vi "X_2.84_Event_Structures.vi"() -> ()   [LabVIEW 2022 SP3]
uses:
  <vilib>/numeric/Random Number (Range) DBL.vi
panel:
  in  "stop":bool
  out "Log":string
  in  "Tab Control":enum32{"Page 1", "Page 2"}(tab)
  in  "Cluster 2":T1
  in  "Cluster":T2
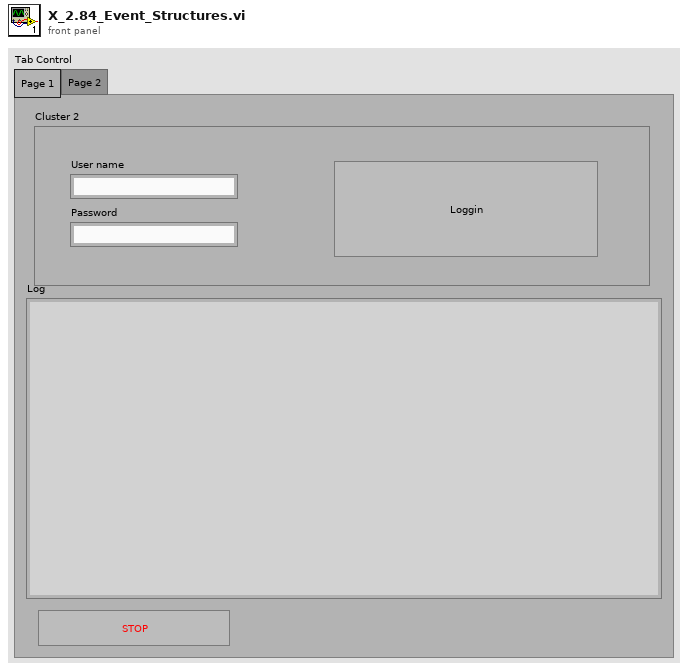
[diagram p1: front panel]
types:
  T1 = cluster{"User name":string, "Password":string, "Loggin":bool}
  T2 = cluster{"Generer Lille":bool, "Generer Stor":bool, "Multiply":bool, "Log af":bool}
  T3 = enum8{"Enabled", "Disabled", "Disabled and Grayed Out"}
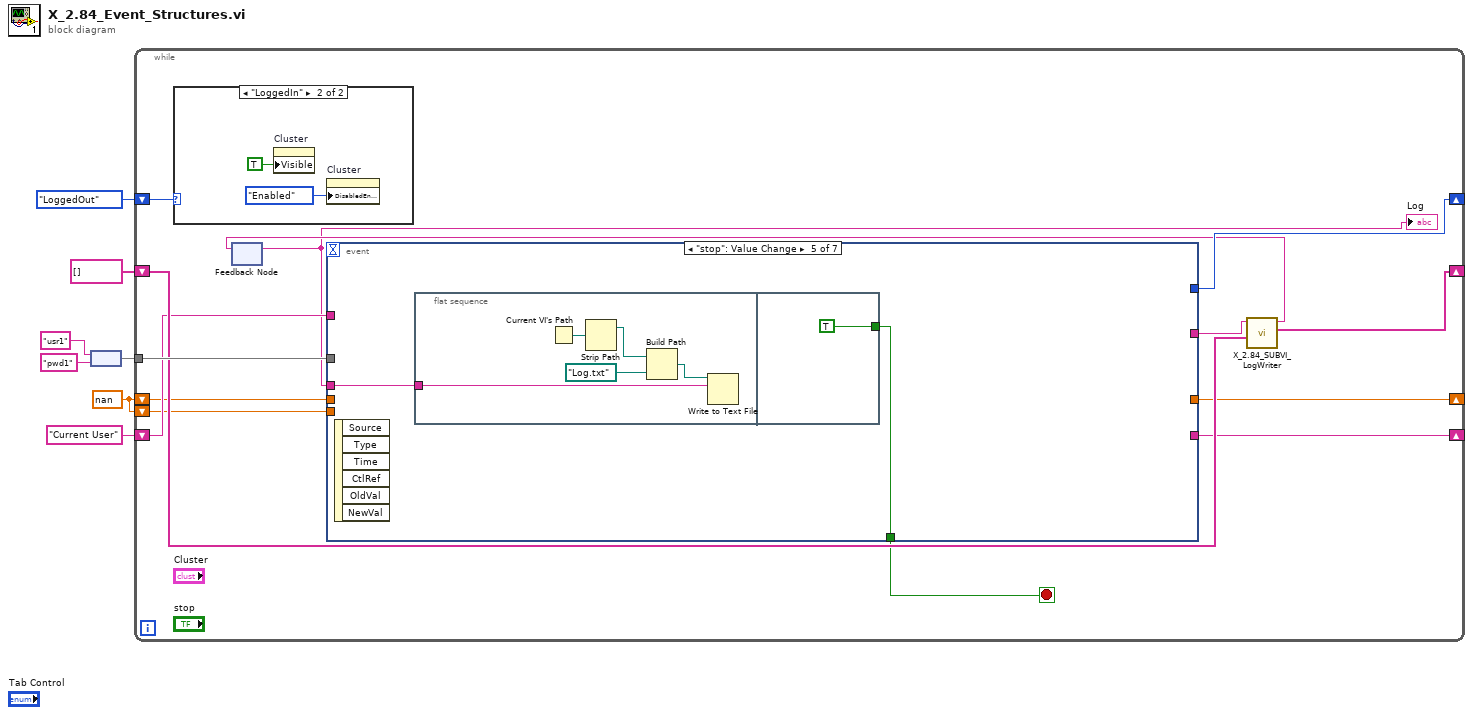
[diagram p0: block diagram]
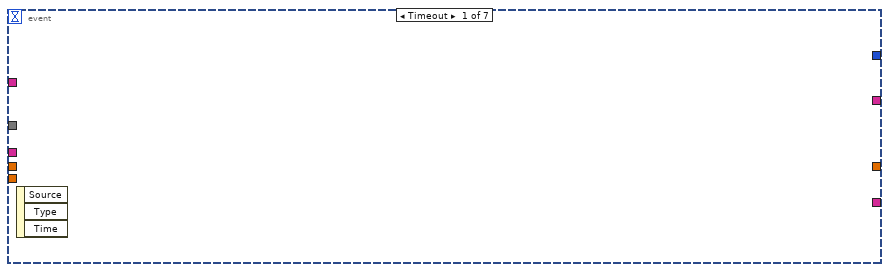
[diagram p2: hidden frame]
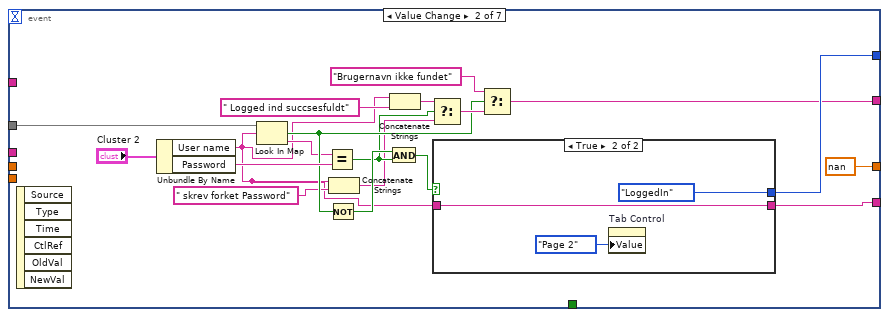
[diagram p3: hidden frame]
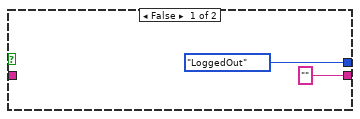
[diagram p4: hidden frame]
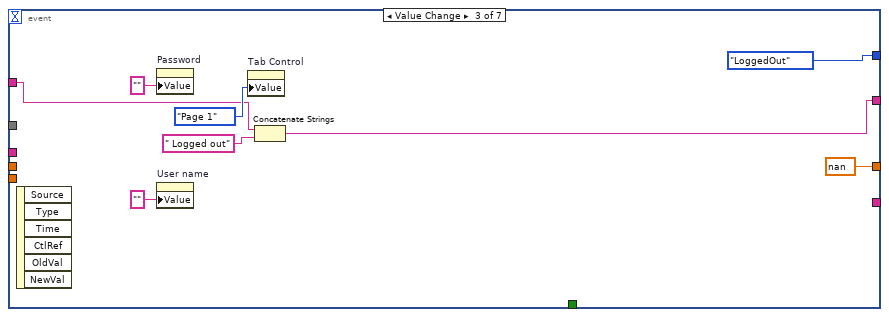
[diagram p5: hidden frame]
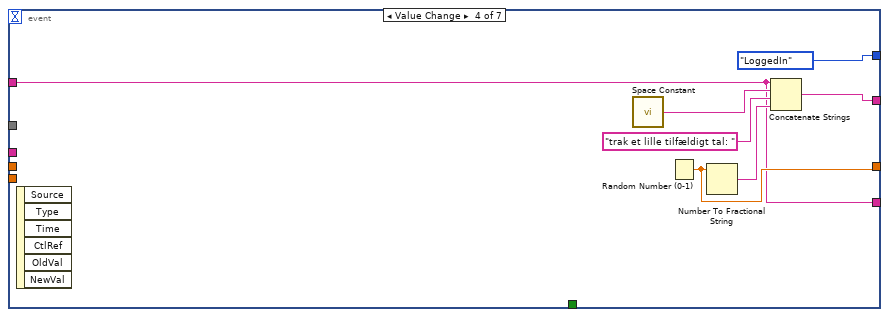
[diagram p6: hidden frame]
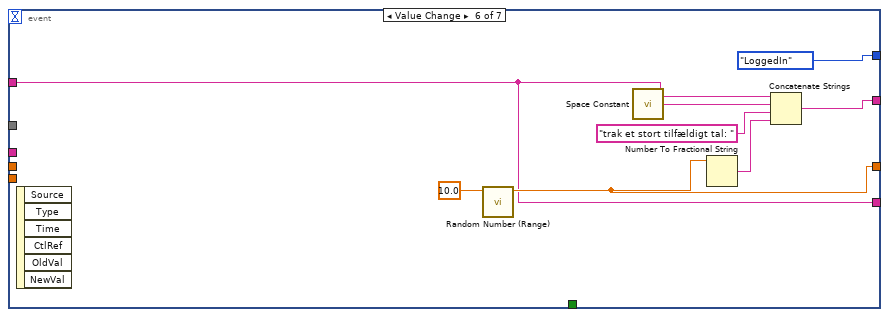
[diagram p7: hidden frame]
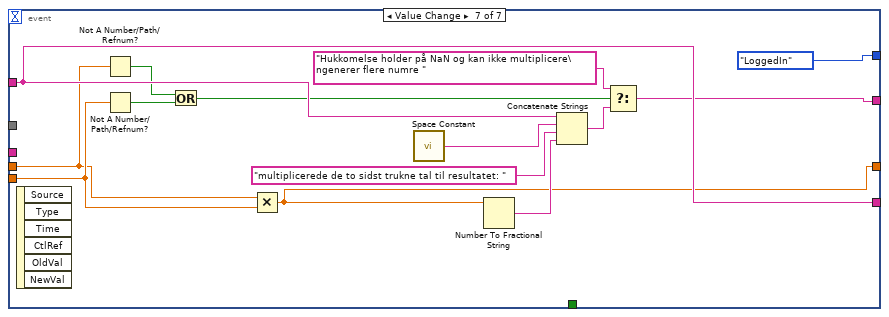
[diagram p8: hidden frame]
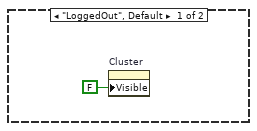
[diagram p9: hidden frame]
diagram:
  w2 = nan
  n1 = node("usr1" ("key"), "pwd1" ("key")) -> (w4:map{string, string})
  n2 = while {
    shift-right: [w19] -> _
    shift-left: enum16{"LoggedOut", "LoggedIn"}."LoggedOut" -> [w20]
    tunnel: w4 -> [w21]
    shift-right: [w17] -> _
    shift-left: string[] [] -> [w18]
    shift-right: [w15] -> _
    shift-left: w2 -> [w11]
    shift-left: w2 -> [w12]
    shift-right: [w14] -> _
    shift-left: "Current User" -> [w13]
    stop <- w10 stop-if-true
    n3 = case shown="\"LoggedIn\"" w20 {
      frame "LoggedOut", Default {
        n4 = property on="Cluster" class="Clust"("Visible"=FALSE) -> ()  [unwired: 2 in, 2 out]
      }
      frame "LoggedIn" {
        n5 = property on="Cluster" class="Clust"("Visible"=TRUE) -> ()  [unwired: 2 in, 2 out]
        n6 = property on="Cluster" class="Clust"("DisabledEnum"=T3."Enabled" ("Disabled")) -> ()  [unwired: 2 in, 2 out]
      }
    }
    n7 = feedback #1() -> (w8:string)  [unwired: 1 in]
    "Log" <- w8
    n8 = event shown="[4] \"stop\": Value Change" {
      selector: _ -> [_ _ _ _ _ _ _]
      dyn-events: _ -> [_ _ _ _ _ _ _]
      timeout: _ -> [_ _ _ _ _ _ _]
      tunnel: w21 -> [_ w40 _ _ _ _ _]
      tunnel: [_ w36 enum16{"LoggedOut", "LoggedIn"}."LoggedOut" enum16{"LoggedOut", "LoggedIn"}."LoggedIn" _ enum16{"LoggedOut", "LoggedIn"}."LoggedIn" enum16{"LoggedOut", "LoggedIn"}."LoggedIn"] -> w19
      tunnel: [_ w35 w46 w55 _ w70 w82] -> w16
      tunnel: [_ nan nan w59 _ w71 w81] -> w15
      tunnel: [_ w29 _ w54 _ w69 w85] -> w14
      tunnel: w13 -> [_ _ w48 w54 _ w69 w85]
      tunnel: w12 -> [_ _ _ _ _ _ w83]
      tunnel: w11 -> [_ _ _ _ _ _ w80]
      tunnel: [_ _ _ _ w62 _ _] -> w10
      tunnel: w8 -> [_ _ _ _ w61 _ _]
      event Timeout {
        n9 = event-data() -> ()  [unwired: 1 in, 3 out]
      }
      event "Cluster 2.Loggin": Value Change {
        n10 = event-data() -> ()  [unwired: 1 in, 6 out]
        n11 = Unbundle By Name("Cluster 2") -> ("User name"=w22:string, "Password"=w39:string)
        n12 = Look In Map(map=w40, key=w22) -> (key not found?=w34:bool, value=w28:string)  [unwired: 1 in]
        n13 = Equal?(x=w28, y=w39) -> (x = y?=w32:bool)
        n14 = Not(x=w34) -> (.not. x?=w33:bool)
        n15 = Concatenate Strings(w22, " skrev forket Password") -> (w25:string)
        n16 = And(x=w33, y=w32) -> (x .and. y?=w31:bool)
        n17 = Concatenate Strings(w22, " Logged ind succsesfuldt") -> (w23:string)
        n18 = Select(t=w23, s=w32, f=w25) -> (s? t:f=w37:string)
        n19 = case shown="True" w31 {
          tunnel: [enum16{"LoggedOut", "LoggedIn"}."LoggedOut" enum16{"LoggedOut", "LoggedIn"}."LoggedIn"] -> w36
          tunnel: w22 -> [_ w43]
          tunnel: ["" ("value") w43] -> w29
          frame False {
          }
          frame True {
            n20 = property on="Tab Control" class="TabCtl (strict)"("Value"=enum32{"Page 1", "Page 2"}."Page 2" ("Tab Control")) -> ()  [unwired: 2 in, 2 out]
          }
        }
        n21 = Select(t="Brugernavn ikke fundet", s=w34, f=w37) -> (s? t:f=w35:string)
      }
      event "Cluster.Log af": Value Change {
        n22 = event-data() -> ()  [unwired: 1 in, 6 out]
        n23 = property on="Password" class="Str"("Value"="") -> ()  [unwired: 2 in, 2 out]
        n24 = property on="User name" class="Str"("Value"="") -> ()  [unwired: 2 in, 2 out]
        n25 = property on="Tab Control" class="TabCtl (strict)"("Value"=enum32{"Page 1", "Page 2"}."Page 1" ("Tab Control")) -> ()  [unwired: 2 in, 2 out]
        n26 = Concatenate Strings(w48, " Logged out") -> (w46:string)
      }
      event "Cluster.Generer Lille": Value Change {
        n27 = event-data() -> ()  [unwired: 1 in, 6 out]
        n28 = call <vilib>:"Space Constant.vi"() -> ("String"=w58:string)
        n29 = Random Number (0-1)() -> (number: 0 to 1=w59:dbl)
        n30 = Number To Fractional String(number=w59) -> (F-format string=w56:string)  [unwired: 3 in]
        n31 = Concatenate Strings(w54, w58, "trak et lille tilfældigt tal: " ("string"), w56) -> (w55:string)
      }
      event "stop": Value Change {
        n32 = event-data() -> ()  [unwired: 1 in, 6 out]
        n33 = flat-sequence {
          tunnel: w61 -> [w66]
          tunnel: [TRUE] -> w62
          frame #0 {
            n34 = Current VI's Path() -> (path=w67:path)
            n35 = Strip Path(path=w67) -> (stripped path=w64:path)  [unwired: 1 out]
            n36 = Build Path(base path=w64, name or relative path=path "Log.txt") -> (appended path=w63:path)
            n37 = Write to Text File(file (use dialog)=w63, text=w66) -> ()  [unwired: 2 in, 3 out]
          }
          frame #1 {
          }
        }
      }
      event "Cluster.Generer Stor": Value Change {
        n38 = event-data() -> ()  [unwired: 1 in, 6 out]
        n39 = call-poly <vilib>:"Random Number (Range).vi"("upper bound (100)"=10.0) -> ("number"=w71:dbl)  [unwired: 10 in]
        n40 = call <vilib>:"Space Constant.vi"() -> ("String"=w76:string)
        n41 = Number To Fractional String(number=w71) -> (F-format string=w74:string)  [unwired: 3 in]
        n42 = Concatenate Strings(w69, w76, "trak et stort tilfældigt tal: " ("string"), w74) -> (w70:string)
      }
      event "Cluster.Multiply": Value Change {
        n43 = event-data() -> ()  [unwired: 1 in, 6 out]
        n44 = Not A Number/Path/Refnum?(number/path/refnum=w80) -> (NaN/Path/Refnum?=w79:bool)
        n45 = Not A Number/Path/Refnum?(number/path/refnum=w83) -> (NaN/Path/Refnum?=w78:bool)
        n46 = Or(x=w79, y=w78) -> (x .or. y?=w77:bool)
        n47 = Multiply(x=w80, y=w83) -> (x*y=w81:dbl)
        n48 = call <vilib>:"Space Constant.vi"() -> ("String"=w88:string)
        n49 = Number To Fractional String(number=w81) -> (F-format string=w86:string)  [unwired: 3 in]
        n50 = Concatenate Strings(w85, w88, "multiplicerede de to sidst trukne tal til resultatet: " ("string"), w86) -> (w84:string)
        n51 = Select(t="Hukkomelse holder på NaN og kan ikke multiplicere\ngenerer flere numre ", s=w77, f=w84) -> (s? t:f=w82:string)
      }
    }
    n52 = call "X_2.84_SUBVI_LogWriter.vi"("Gen goende array ind"=w18, "Ny string"=w16) -> ("Gen goende aray out"=w17:string[], "Log out"=w9:string)  [unwired: 8 in]
    n53 = feedback-in #1(w9) -> ()
  }
